vi "Interconvert SGL and Variant Arrays.vi"(0 "SGL 1D Array In":sgl[](array[numeric]) format="%.2f", 5 "SGL 1D Array 2 In":sgl[](array[numeric]) format="%.2f", 7 "SGL 2D Array In":sgl[][](array[numeric]) format="%.2f", 9 "Variant 1D Array In":variant[](array[variant]), 11 "Variant 2D Array In":variant[][](array[variant])) -> (4 "Variant 1D Array Out":variant[](array[variant]), 6 "Variant 1D Array 2 Out":variant[](array[variant]), 8 "Variant 2D Array Out":variant[][](array[variant]), 10 "SGL 1D Array Out":sgl[](array[numeric]) format="%.2f", 15 "SGL 2D Array Out":sgl[][](array[numeric]) format="%.2f")   [LabVIEW 2009]
doc: "This VI interconverts 1D and 2D arrays between single-precision floating point numbers and variants.\n\nCoded by Douglas A. Femec, January 24, 2006.\n\nCopyright (c) 2006 MKS Instruments, Inc.\nAll rights reserved."
panel:
  # "Copyright (c) 2006 MKS Instruments, Inc.\nAll rights reserved."
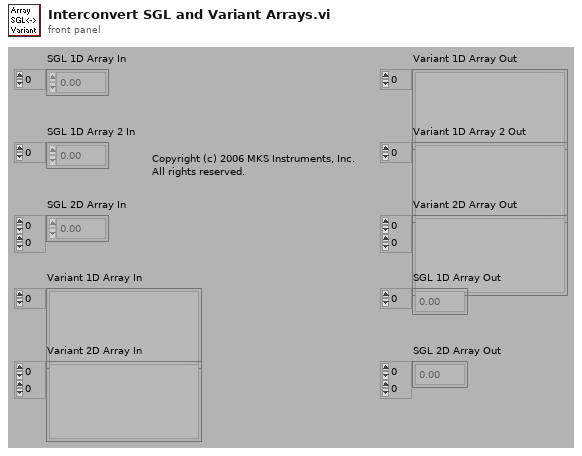
[diagram p1: front panel]
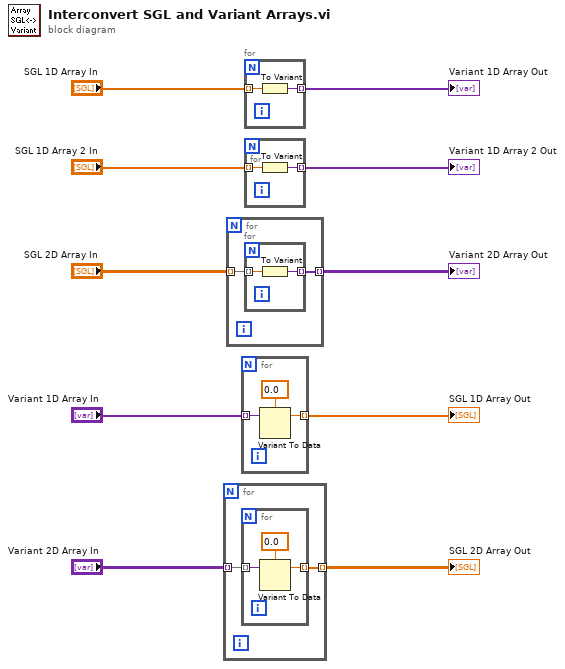
[diagram p0: block diagram]
diagram:
  n1 = for {
    tunnel: "Variant 2D Array In" -> [w12] mode=indexing
    tunnel: [w11] -> w1 mode=indexing
    n2 = for {
      tunnel: [w15] -> w11 mode=indexing
      tunnel: w12 -> [w14] mode=indexing
      n3 = Variant To Data(Variant=w14, type=sgl 0.0) -> (data=w15:sgl)  [unwired: 1 in, 1 out]
    }
  }
  "SGL 2D Array Out" <- w1
  n4 = for {
    tunnel: "SGL 2D Array In" -> [w17] mode=indexing
    tunnel: [w16] -> w5 mode=indexing
    n5 = for {
      tunnel: w17 -> [w19] mode=indexing
      tunnel: [w18] -> w16 mode=indexing
      n6 = To Variant(anything=w19) -> (Variant=w18:variant)
    }
  }
  "Variant 2D Array Out" <- w5
  n7 = for {
    tunnel: [w22] -> w3 mode=indexing
    tunnel: "Variant 1D Array In" -> [w21] mode=indexing
    n8 = Variant To Data(Variant=w21, type=sgl 0.0) -> (data=w22:sgl)  [unwired: 1 in, 1 out]
  }
  "SGL 1D Array Out" <- w3
  n9 = for {
    tunnel: "SGL 1D Array In" -> [w24] mode=indexing
    tunnel: [w23] -> w9 mode=indexing
    n10 = To Variant(anything=w24) -> (Variant=w23:variant)
  }
  "Variant 1D Array Out" <- w9
  n11 = for {
    tunnel: "SGL 1D Array 2 In" -> [w26] mode=indexing
    tunnel: [w25] -> w8 mode=indexing
    n12 = To Variant(anything=w26) -> (Variant=w25:variant)
  }
  "Variant 1D Array 2 Out" <- w8
